vi "Analisis de Fourier.vi"() -> ()   [LabVIEW 2014]
uses:
  <vilib>/express/express analysis/Spectral/Block/exnSpectralBlock spectral measurements RMS poly.vi
  <vilib>/express/express analysis/Spectral/Block/exnSpectralBlock spectral measurements RMS WFM.vi
  <vilib>/express/express analysis/Spectral/XNode/ExpressSpectralMeasurementsBlockNode.xnode
  <vilib>/measure/NI_MABase.lvlib
panel:
  out "SIgnal":waveform(dbl)(graph)
  out "Fourier":cluster{"f0":dbl, "df":dbl, "magnitude":dbl[]}(graph)
  in  "Duty Cycle":dbl(slide) scale=0.0..100.0
  in  "Enum":T1(ring)
  in  "Amplitude":dbl(knob) scale=0.0..20.0
  in  "x1":dbl(slide) scale=0.0..9.0
  in  "x10":dbl(slide) scale=0.0..90.0
  in  "x100":dbl(slide) scale=0.0..4.0
  # "x1"
  # "x100"
  # "x10"
  # "HERTZ"
  # "Tipo de Senal"
  # "Amplitude"
  # "Duty Cycle"
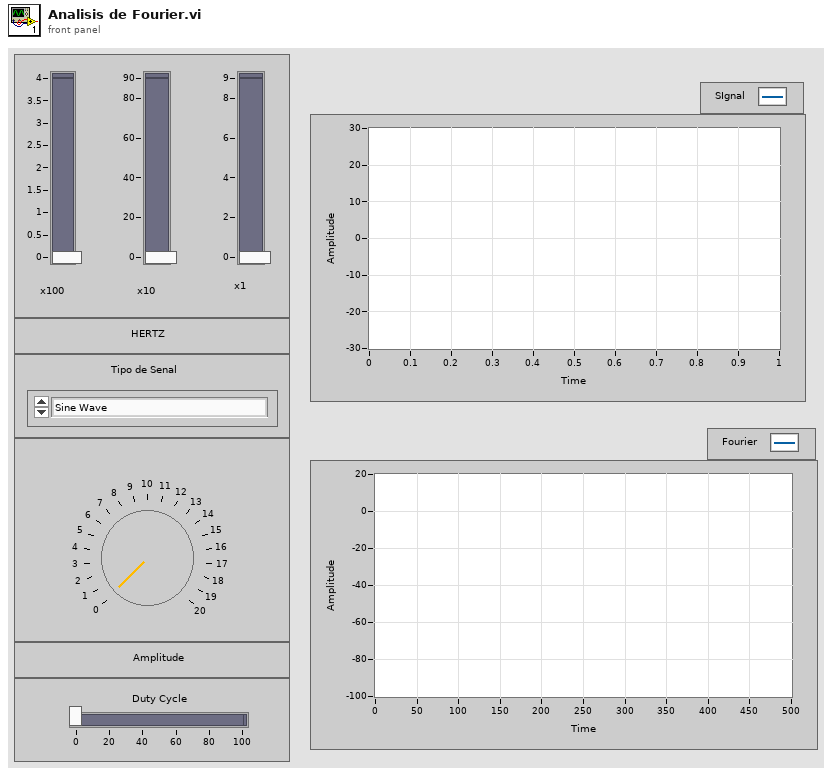
[diagram p1: front panel]
types:
  T1 = enum16{"Sine Wave", "Triangle Wave", "Square Wave", "Sawtooth Wave"}
  T2 = cluster{"averaging mode":u16, "weighting mode":u16, "number of averages":u32}
  T3 = cluster{"dB On (F)":bool, "unwrap phase (F)":bool, "convert to degree (F)":bool}
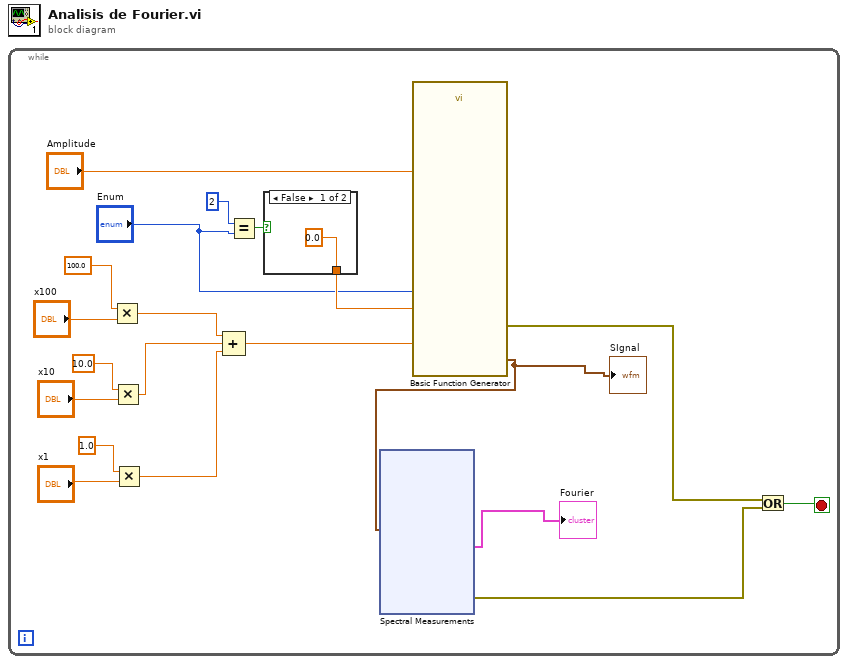
[diagram p0: block diagram]
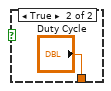
[diagram p2: hidden frame]
diagram:
  n1 = while {
    stop <- w5 stop-if-true
    n2 = Multiply(x=100.0, y="x100") -> (x*y=w12:dbl)
    n3 = Multiply(x=10.0, y="x10") -> (x*y=w13:dbl)
    n4 = Multiply(x=1.0, y="x1") -> (x*y=w14:dbl)
    n5 = Compound Arithmetic op=ADD(w12, w13, w14) -> (w11:dbl)
    n6 = Equal?(x=u16 2, y="Enum") -> (x = y?=w8:bool)
    n7 = case shown="False" w8 {
      tunnel: [0.0 "Duty Cycle"] -> w9
      frame False {
      }
      frame True {
      }
    }
    n8 = call <vilib>:"Basic Function Generator.vi"("square wave duty cycle (%)"=w9, "signal type"="Enum", "amplitude"="Amplitude", "frequency"=w11) -> ("error out"=w4:errorcluster, "signal out"=w1:waveform(dbl))  [unwired: 5 in, 1 out]
    "SIgnal" <- w1
    n9 = xnode "Spectral Measurements"("Signals"=w1) -> ("FFT - (RMS)"=→"Fourier":cluster{"f0":dbl, "df":dbl, "magnitude":dbl[]}, "error out"=w3:errorcluster)  [unwired: 1 in, 1 out]
    n10 = Or(x=w4, y=w3) -> (x .or. y?=w5:bool)
  }
